vi "ClusterToString.vi"(8 "Error in (no error)":errorcluster, 11 "Cluster":variant) -> (0 "Error out":errorcluster, 3 "String out":string)   [LabVIEW 2011]
doc: "Use this VI to change any data into a string."
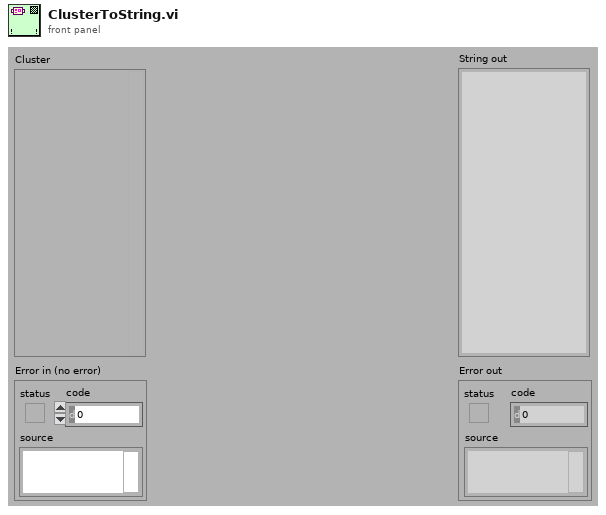
[diagram p1: front panel]
types:
  T1 = typedef "Type Descriptor Header__ogtk.ctl" = cluster{"length":u16, "private":u8, "type":T2, "# elements":u16}
  T2 = typedef "Type Descriptor Enumeration__ogtk.ctl" = enum8{"<Null>", "I8", "I16", "I32", "I64", "U8", "U16", "U32", "U64", "SGL", "DBL", "EXT", "CSG", "CDB", "CXT", "0x0F", "0x10", "0x11", "0x12", "0x13", "0x14", "Enum U8", "Enum U16", "Enum U32", "Enum U64", "SGL PQ", "DBL PQ", "EXT PQ", "CSG PQ", "CDB PQ", "CXT PQ", "0x1F", "0x20", "Boolean", "0x22", "0x23", "0x24", "0x25", "0x26", "0x27", "0x28", "0x29", "0x2A", "0x2B", "0x2C", "0x2D", "0x2E", "0x2F", "String", "0x31", "Path", "Pict", "0x34", "0x35", "0x36", "DAQ", "0x38", "0x39", "0x3A", "0x3B", "0x3C", "0x3D", "0x3E", "0x3F", "Array", "0x41", "0x42", "0x43", "0x44", "0x45", "0x46", "0x47", "0x48", "0x49", "0x4A", "0x4B", "0x4C", "0x4D", "0x4E", "0x4F", "Cluster", "0x51", "0x52", "Variant", "Waveform", "0x55", "0x56", "0x57", "0x58", "0x59", "0x5A", "0x5B", "0x5C", "0x5D", "0x5E", "0x5F", "0x60", "0x61", "0x62", "0x63", "0x64", "0x65", "0x66", "0x67", "0x68", "0x69", "0x6A", "0x6B", "0x6C", "0x6D", "0x6E", "0x6F", "Refnum"}
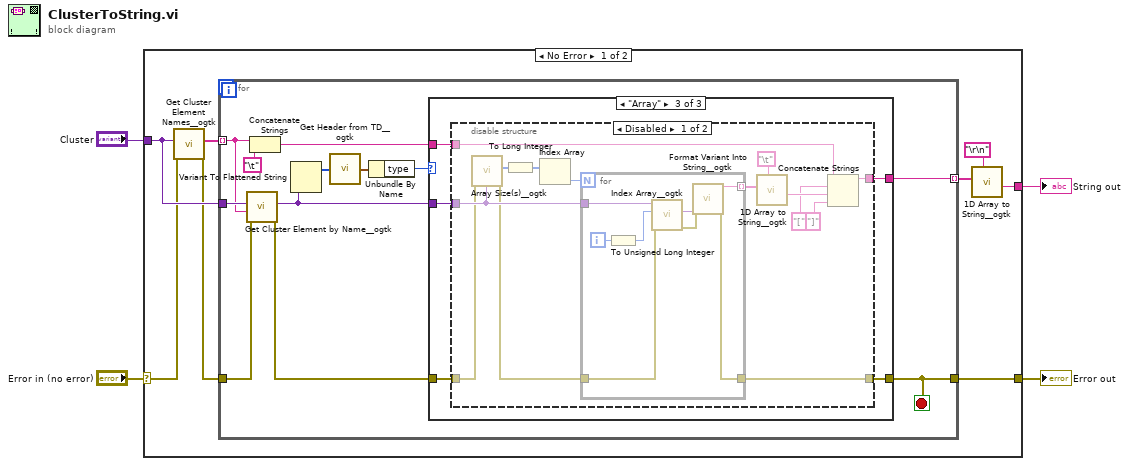
[diagram p0: block diagram]
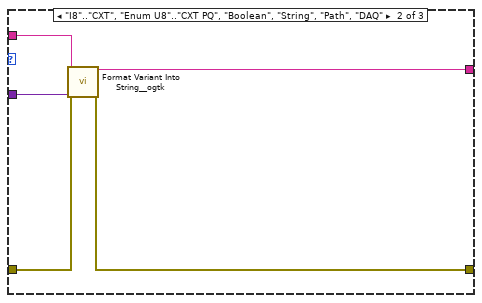
[diagram p3: hidden frame]
diagram:
  n1 = case shown="No Error" "Error in (no error)" {
    selector: "Error in (no error)" -> [w8 w59]
    tunnel: [w11 w59] -> w2
    tunnel: "Cluster" -> [w10 _]
    tunnel: [w5 _] -> w4
    frame No Error {
      n2 = call <userlib>:"Get Cluster Element Names__ogtk.vi"("error in (no error)"=w8, "Cluster"=w10) -> ("error out"=w9:errorcluster, "Element Names"=w12:string[])  [unwired: 8 in]
      n3 = for {
        tunnel: w12 -> [w22] mode=indexing
        tunnel: w10 -> [w24]
        tunnel: [w13] -> w7 mode=indexing
        tunnel: w9 -> [w21]
        tunnel: [w14] -> w11
        stop <- w14 stop-if-true
        n4 = call <userlib>:"Get Cluster Element by Name__ogtk.vi"("error in (no error)"=w21, "Element Name"=w22, "Cluster"=w24) -> ("error out"=w15:errorcluster, "VElement"=w16:variant)  [unwired: 6 in, 1 out]
        n5 = Concatenate Strings(w22, "\t") -> (w17:string)
        n6 = Variant To Flattened String(Variant=w16) -> (1:w20:i16[])  [unwired: 1 out]
        n7 = call <userlib>:"Get Header from TD__ogtk.vi"("Type Descriptor"=w20) -> ("Type Descriptor Header"=w19:T1)
        n8 = Unbundle By Name(w19) -> ("type"=w18:T2)
        n9 = case shown="\"Array\"" w18 {
          tunnel: w17 -> [_ w30 w31]
          tunnel: w16 -> [_ w29 w35]
          tunnel: w15 -> [w25 w28 w33]
          tunnel: [w25 w27 w34] -> w14
          tunnel: [_ w26 w32] -> w13
          frame "<Null>", Default {
            # "Error"
          }
          frame "I8".."CXT", "Enum U8".."CXT PQ", "Boolean", "String", "Path", "DAQ" {
            n10 = call <userlib>:"Format Variant Into String__ogtk.vi"("Input String"=w30, "error in (no error)"=w28, "Variant"=w29) -> ("Output String"=w26:string, "error out"=w27:errorcluster)  [unwired: 11 in]
          }
          frame "Array" {
            n11 = disable-structure shown="Disabled" {
              disable-tunnel: w35 -> [w46 _]
              disable-tunnel: [w45 w58] -> w34
              disable-tunnel: w33 -> [w44 w58]
              disable-tunnel: [w38 _] -> w32
              disable-tunnel: w31 -> [w37 _]
              frame Disabled {
                n12 = call <userlib>:"Array Size(s)__ogtk.vi"("error in (no error)"=w44, "Array"=w46) -> ("error out"=w36:errorcluster, "Size(s)"=w49:u32[])  [unwired: 7 in, 1 out]
                n13 = To Long Integer(number=w49) -> (32bit integer=w47:i32[])
                n14 = Index Array(array=w47) -> (element=w48:i32)  [unwired: 1 in]
                n15 = for {
                  N: w48 -> [_]
                  tunnel: w46 -> [w57]
                  tunnel: [w52] -> w45
                  tunnel: w36 -> [w54]
                  tunnel: [w50] -> w43 mode=indexing
                  i -> [w56]
                  n16 = To Unsigned Long Integer(number=w56) -> (unsigned 32bit integer=w51:u32)
                  n17 = call <userlib>:"Index Array__ogtk.vi"("error in (no error)"=w54, "Index (1D)"=w51, "MultiD Array"=w57) -> ("error out"=w53:errorcluster, "Array Element"=w55:variant)  [unwired: 7 in]
                  n18 = call <userlib>:"Format Variant Into String__ogtk.vi"("error in (no error)"=w53, "Variant"=w55) -> ("Output String"=w50:string, "error out"=w52:errorcluster)  [unwired: 12 in]
                }
                n19 = call <userlib>:"1D Array to String__ogtk.vi"("delimiter (Tab)"="\t", "Array of Strings"=w43) -> ("delimited string"=w41:string)  [unwired: 9 in]
                n20 = Concatenate Strings(w37, "[" ("string"), w41, "]" ("string")) -> (w38:string)
              }
              frame Enabled {
                # "Not sure if I should support this,\nfor now just throw a error"
              }
            }
          }
        }
      }
      n21 = call <userlib>:"1D Array to String__ogtk.vi"("delimiter (Tab)"="\r\n", "Array of Strings"=w7) -> ("delimited string"=w5:string)  [unwired: 9 in]
    }
    frame Error {
    }
  }
  "Error out" <- w2
  "String out" <- w4
